vi "Clean Up Structures.vi"(8 "error in (no error)":errorcluster, 11 "Block Diagram in":refnum<class "VI.lvclass">) -> (0 "error out":errorcluster, 3 "Block Diagram out":refnum<class "VI.lvclass">)   [LabVIEW 2015, in "VI.lvclass"]
uses:
  VI.lvclass
  VI.lvclass/VI.ctl
  Module Loop/Read Modules.vi
  Module/Module/Module.lvclass
  Loop/Loop.lvclass
  Main Sequence/Main Sequence.lvclass
  Module Loop/Module Loop.lvclass
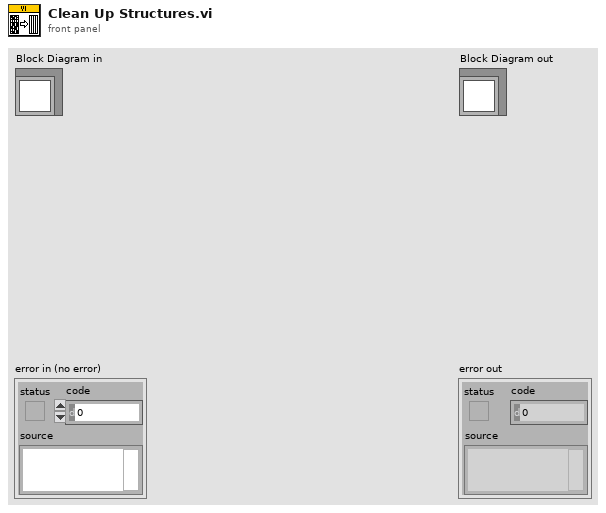
[diagram p1: front panel]
types:
  T1 = enum32{"Top Edges", "Vertical Centers", "Bottom Edges", "Vertical Gap", "Vertical Compress", "Left Edges", "Horizontal Centers", "Right Edges", "Horizontal Gap", "Horizontal Compress"}
  T2 = enum32{"Top Edges", "Vertical Centers", "Bottom Edges", "Left Edges", "Horizontal Centers", "Right Edges"}
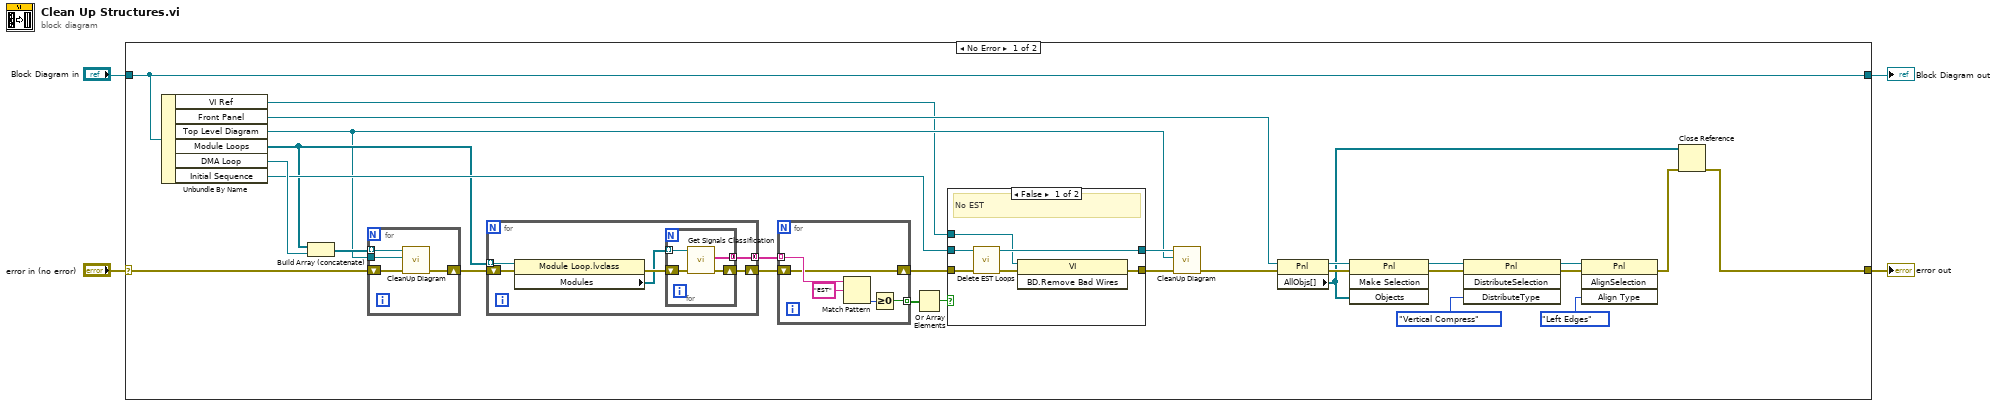
[diagram p0: block diagram]
diagram:
  n1 = case shown="No Error" "error in (no error)" {
    selector: "error in (no error)" -> [w12 w62]
    tunnel: [w20 w62] -> w3
    tunnel: [w33 w61] -> w1
    tunnel: "Block Diagram in" -> [w33 w61]
    frame No Error {
      n2 = Unbundle By Name(w33) -> ("VI Ref"=w5:refnum<vi>, "Front Panel"=w30:refnum<vi>, "Top Level Diagram"=w7:refnum<vi>, "Module Loops"=w11:refnum<class "Module Loop.lvclass">[], "DMA Loop"=w32:refnum<class "DMA Loop.lvclass">, "Initial Sequence"=w14:refnum<class "Main Sequence.lvclass">)
      n3 = Build Array (concatenate)(w11, w32) -> (w31:refnum<class "Loop.lvclass">[])
      n4 = for {
        tunnel: w31 -> [w60] mode=indexing
        tunnel: w7 -> [w59]
        shift-right: [w57] -> w13
        shift-left: w12 -> [w58]
        n5 = call-dynamic "CleanUp Diagram.vi"("error in (no error)"=w58, "Top Level Diagram"=w59, "Loop in"=w60) -> ("error out"=w57:errorcluster)  [unwired: 7 in, 1 out]
      }
      n6 = for {
        shift-right: [w52] -> w17
        shift-left: w13 -> [w50]
        tunnel: w11 -> [w51] mode=indexing
        tunnel: [w47] -> w18 mode=concatenating
        n7 = property class="Module Loop.lvclass"(reference=w51, error in=w50) -> (error out=w49:errorcluster, "Modules"=w48:refnum<class "Module.lvclass">[])  [unwired: 1 out]
        n8 = for {
          shift-right: [w55] -> w52
          shift-left: w49 -> [w56]
          tunnel: w48 -> [w54] mode=indexing
          tunnel: [w53] -> w47 mode=concatenating
          n9 = call "Get Signals Classification.vi"("error in (no error)"=w56, "Module in"=w54) -> ("error out"=w55:errorcluster, "Classifications"=w53:string[])  [unwired: 7 in, 1 out]
        }
      }
      n10 = for {
        tunnel: w18 -> [w46] mode=indexing
        shift-right: [w44] -> w10
        shift-left: w17 -> [w44]
        tunnel: [w42] -> w16 mode=indexing
        n11 = Match Pattern(string=w46, regular expression="EST") -> (offset past match=w43:i32)  [unwired: 1 in, 3 out]
        n12 = Greater Or Equal To 0?(x=w43) -> (x >= 0?=w42:bool)
      }
      n13 = Or Array Elements(Boolean array=w16) -> (logical OR=w15:bool)
      n14 = case shown="False" w15 {
        tunnel: w10 -> [w39 w41]
        tunnel: [w35 w41] -> w6
        tunnel: w14 -> [w38 w40]
        tunnel: [w37 w40] -> w8
        tunnel: w5 -> [w34 _]
        frame False {
          # "No EST"
          n15 = call "Delete EST Loops.vi"("error in (no error)"=w39, "Main Sequence in"=w38) -> ("error out"=w36:errorcluster, "Main Sequence out"=w37:refnum<class "Main Sequence.lvclass">)  [unwired: 8 in]
          n16 = invoke class="VI" method="BD.Remove Bad Wires"(reference=w34, error in=w36) -> (error out=w35:errorcluster)  [unwired: 1 in, 2 out]
        }
        frame True {
        }
      }
      n17 = call-dynamic "CleanUp Diagram.vi"("error in (no error)"=w6, "Top Level Diagram"=w7, "Initial Sequence in"=w8) -> ("error out"=w9:errorcluster)  [unwired: 7 in, 1 out]
      n18 = property class="Pnl"(reference=w30, error in=w9) -> (reference out=w29:refnum<vi>, error out=w28:errorcluster, "AllObjs[]"=w19:refnum<vi>[])
      n19 = invoke class="Pnl" method="Make Selection"(reference=w29, error in=w28, "Objects"=w19) -> (reference out=w26:refnum<vi>, error out=w25:errorcluster)  [unwired: 1 in, 2 out]
      n20 = invoke class="Pnl" method="DistributeSelection"(reference=w26, error in=w25, "DistributeType"=T1."Vertical Compress") -> (reference out=w24:refnum<vi>, error out=w23:errorcluster)  [unwired: 1 in, 2 out]
      n21 = invoke class="Pnl" method="AlignSelection"(reference=w24, error in=w23, "Align Type"=T2."Left Edges") -> (error out=w21:errorcluster)  [unwired: 1 in, 3 out]
      n22 = Close Reference(reference=w19, error in (no error)=w21) -> (error out=w20:errorcluster)
    }
    frame Error {
    }
  }
  "error out" <- w3
  "Block Diagram out" <- w1
